vi "Initialize.vi"(5 "Baud Rate (115200)":T1=115200 items=["9600"=9600, "19200"=19200, "28800"=28800, "115200"=115200], 7 "timeout (500ms)":u32=10000, 8 "error in (no error)":errorcluster, 11 "VISA resource name":refnum<visa-resource-name>) -> (0 "error out":errorcluster, 3 "VISA resource name out":refnum<visa-resource-name>)   [LabVIEW 2018, in "ASI TG-1000.lvlib"]
doc: "Establishes communication with the instrument and optionally performs an instrument identification query and/or an instrument reset. It also places the instrument in a default state needed for other instrument driver operations. Therefore, call this VI before calling other instrument driver VIs for this instrument. Generally, you need to call the Initialize VI only once at the beginning of an application."
uses:
  ASI TG-1000.lvlib
  Utility/Baud Rate.ctl
  <vilib>/Instr/_visa.llb/VISA Configure Serial Port (Instr).vi
panel:
  # "(c) 2014 Applied Scientific Insturmentation. ALL RIGHTS RESERVED."
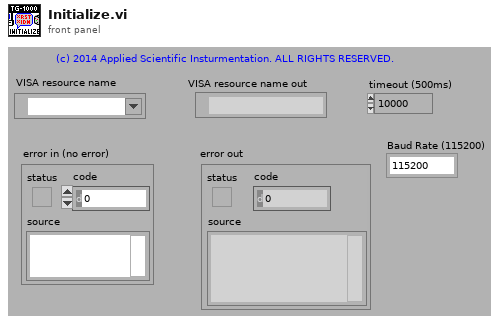
[diagram p1: front panel]
types:
  T1 = typedef "ASI TG-1000.lvlib/Baud Rate.ctl" = u32
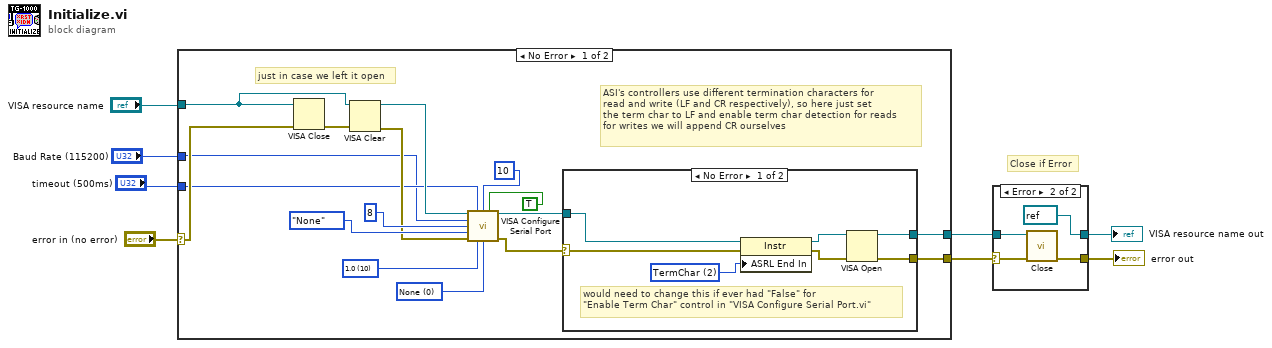
[diagram p0: block diagram]
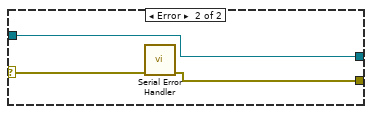
[diagram p2: hidden frame]
diagram:
  # "Close if Error"
  n1 = case shown="No Error" "error in (no error)" {
    selector: "error in (no error)" -> [w15 w37]
    tunnel: "VISA resource name" -> [w12 w36]
    tunnel: [w18 w37] -> w4
    tunnel: [w17 w36] -> w3
    tunnel: "timeout (500ms)" -> [w10 _]
    tunnel: "Baud Rate (115200)" -> [w9 _]
    frame No Error {
      w21 = u16 0 items=["None", "XON/XOFF", "RTS/CTS", "XON/XOFF & RTS/CTS", "DTR/DSR", "XON/XOFF & DTR/DSR"] ("flow control (0:none)")
      w22 = u16 10 items=["1.0"=10, "1.5"=15, "2.0"=20] ("stop bits (10: 1 bit)")
      # "just in case we left it open"
      # "ASI's controllers use different termination characters for\nread and write (LF and CR respectively), so here just set\nthe term char to LF and enable term char detection for reads\nfor writes we will append CR ourselves"
      n2 = VISA Close(VISA resource name=w12, error in (no error)=w15) -> (error out=w14:errorcluster)
      n3 = VISA Clear(VISA resource name=w12, error in (no error)=w14) -> (VISA resource name out=w11:refnum<visa-resource-name>, error out=w13:errorcluster)
      n4 = call-poly "VISA Configure Serial Port"("VISA resource name"=w11, "timeout (10sec)"=w10, "termination char\n(0xA = '\\n' = LF)"=u8 10 ("termination char\n(0xA = '\\n' = LF)"), "Enable Termination\nChar (T)"=TRUE ("Enable Termination\nChar (T)"), "baud rate (9600)"=w9, "data bits (8)"=u16 8, "parity (0:none)"=enum16{"None", "Odd", "Even", "Mark", "Space"}."None", "error in (no error)"=w13, "stop bits (10: 1 bit)"=w22, "flow control (0:none)"=w21) -> ("VISA resource name out"=w19:refnum<visa-resource-name>, "error out"=w16:errorcluster)  [unwired: 4 in]
      n5 = case shown="No Error" w16 {
        selector: w16 -> [w26 w34]
        tunnel: w19 -> [w31 w35]
        tunnel: [w30 w33] -> w18
        tunnel: [w27 w35] -> w17
        frame No Error {
          w32 = u16 2 items=["None", "Last Bit", "TermChar"] ("Serial Settings:End Mode for Reads")
          # "would need to change this if ever had \"False\" for\n\"Enable Term Char\" control in \"VISA Configure Serial Port.vi\""
          n6 = property class="Instr"(reference=w31, error in=w26, "ASRL End In"=w32) -> (reference out=w28:refnum<visa-resource-name>, error out=w29:errorcluster)
          n7 = VISA Open(error in (no error)=w29, VISA resource name=w28) -> (VISA resource name=w27:refnum<visa-resource-name>, error out=w30:errorcluster)  [unwired: 3 in]
        }
        frame Error {
          n8 = call "Serial Error Handler.vi"("error in (no error)"=w34) -> ("error out"=w33:errorcluster)  [unwired: 10 in]
        }
      }
    }
    frame Error {
    }
  }
  n9 = case shown="Error" w4 {
    selector: w4 -> [w39 w42]
    tunnel: [w38 refnum<visa-resource-name> refnum ("VISA resource name out")] -> w8
    tunnel: [w39 w43] -> w7
    tunnel: w3 -> [w38 w40]
    frame No Error {
    }
    frame Error {
      n10 = call "Close.vi"("error in (no error)"=w42, "VISA resource name"=w40) -> ("error out"=w43:errorcluster)  [unwired: 9 in]
    }
  }
  "VISA resource name out" <- w8
  "error out" <- w7
